vi "VIPM_Remove Path Duplicates.vi"(11 "Package Array in":T1[](array[typedef])) -> (3 "Package Array out":T1[](array[typedef]))   [LabVIEW 2019]
doc: "Remove paths that are found more than once as these are non unique and cannot be used as identifiers."
uses:
  3e4cba3d-6ed9-4f99-bdc5-95ba8687fde4.vi
  Ctl/Ctl_Package Identifier Cluster.ctl
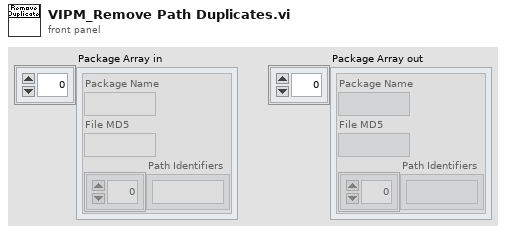
[diagram p1: front panel]
types:
  T1 = typedef "Ctl_Package Identifier Cluster.ctl" = cluster{"Package Name":string, "File MD5":string, "Path Identifiers":string[]}
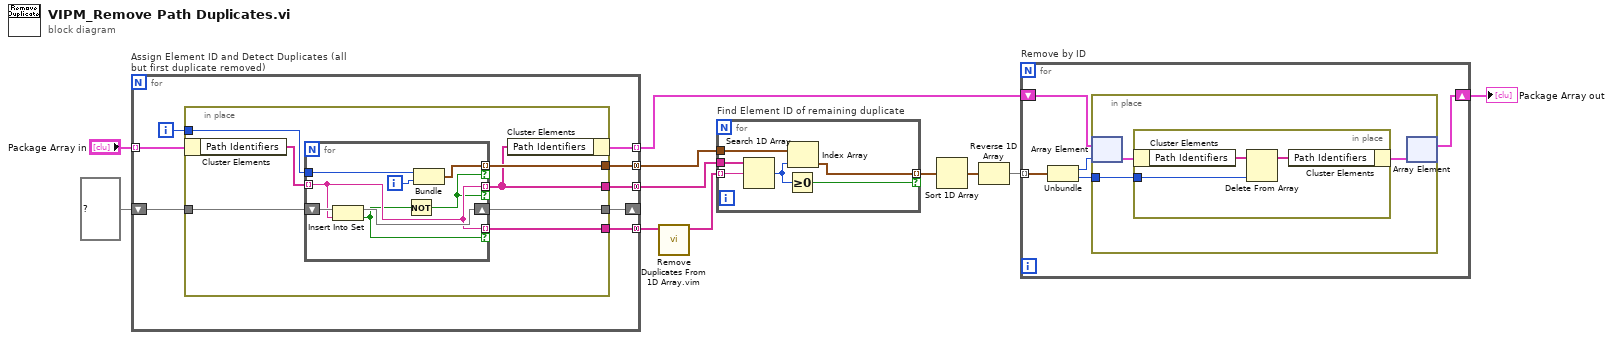
[diagram p0: block diagram]
diagram:
  n1 = for "Assign Element ID and Detect Duplicates (all but first duplicate removed)" {
    tunnel: "Package Array in" -> [w17] mode=indexing
    shift-right: [w13] -> _
    shift-left: set{string} {} ("set") -> [w18]
    tunnel: [w16] -> w3 mode=indexing
    tunnel: [w15] -> w6 mode=concatenating
    tunnel: [w14] -> w9 mode=concatenating
    tunnel: [w12] -> w8 mode=concatenating
    i -> [w19]
    n2 = in-place {
      in-place-border: w19 -> [w26]
      in-place-border: w18 -> [w25]
      in-place-border: [w23] -> w15
      in-place-border: [w22] -> w14
      in-place-border: [w21] -> w13
      in-place-border: [w20] -> w12
      n3 = in-place-cluster #1(w17) -> ("Path Identifiers"=w24:string[])
      n4 = for {
        tunnel: w24 -> [w29] mode=indexing
        tunnel: [w29] -> w20 mode=indexing if=w27
        tunnel: w26 -> [w33]
        tunnel: [w32] -> w23 mode=indexing if=w27
        shift-right: [w30] -> w21
        shift-left: w25 -> [w31]
        tunnel: [w29] -> w22 mode=indexing if=w28
        i -> [w34]
        n5 = Insert Into Set(10:w29, 11:w31) -> (2:w28:bool, 3:w30:set{string})
        n6 = Not(x=w28) -> (.not. x?=w27:bool)
        n7 = Bundle(w33, w34) -> (w32:cluster{i32, i32})  [unwired: 1 in]
      }
      n8 = in-place-cluster #1("Path Identifiers"=w20) -> (w16:T1)
    }
  }
  n9 = call "Remove Duplicates From 1D Array.vim"("array"=w9) -> ("array with duplicates removed"=w7:string[])  [unwired: 10 in]
  n10 = for "Find Element ID of remaining duplicate" {
    tunnel: w8 -> [w40]
    tunnel: w7 -> [w39] mode=indexing
    tunnel: w6 -> [w38]
    tunnel: [w36] -> w5 mode=indexing if=w35
    n11 = Search 1D Array(1D array=w40, element=w39) -> (index of element=w37:i32)  [unwired: 1 in]
    n12 = Greater Or Equal To 0?(x=w37) -> (x >= 0?=w35:bool)
    n13 = Index Array(array=w38, index=w37) -> (element=w36:cluster{i32, i32})
  }
  n14 = Sort 1D Array(array=w5) -> (sorted array=w4:cluster{i32, i32}[])
  n15 = Reverse 1D Array(array=w4) -> (reversed array=w2:cluster{i32, i32}[])
  n16 = for "Remove by ID" {
    shift-right: [w41] -> w1
    shift-left: w3 -> [w44]
    tunnel: w2 -> [w45] mode=indexing
    n17 = Unbundle(w45) -> (w43:i32, w42:i32)
    n18 = in-place {
      in-place-border: w42 -> [w47]
      n19 = in-place-array #2(w44, w43) -> (w48:T1)
      n20 = in-place {
        in-place-border: w47 -> [w50]
        n21 = in-place-cluster #3(w48) -> ("Path Identifiers"=w51:string[])
        n22 = Delete From Array(array=w51, index=w50) -> (array with subset deleted=w49:string[])  [unwired: 1 in, 1 out]
        n23 = in-place-cluster #3("Path Identifiers"=w49) -> (w46:T1)
      }
      n24 = in-place-array #2(w46) -> (w41:T1[])  [unwired: 1 out]
    }
  }
  "Package Array out" <- w1
